vi "非均匀ADC.vi"(0 "输入的模拟信号取样值 V":dbl=2.56, 3 "Vref V":dbl=2.56) -> (7 "数字编码":i32[](array[numeric]))   [LabVIEW 2020]
panel:
  out "Numeric":i32
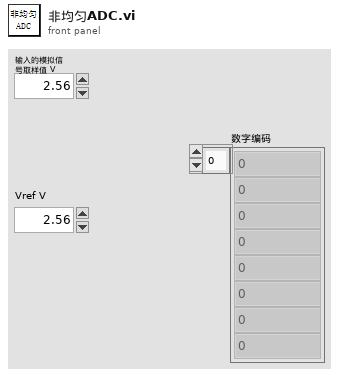
[diagram p1: front panel]
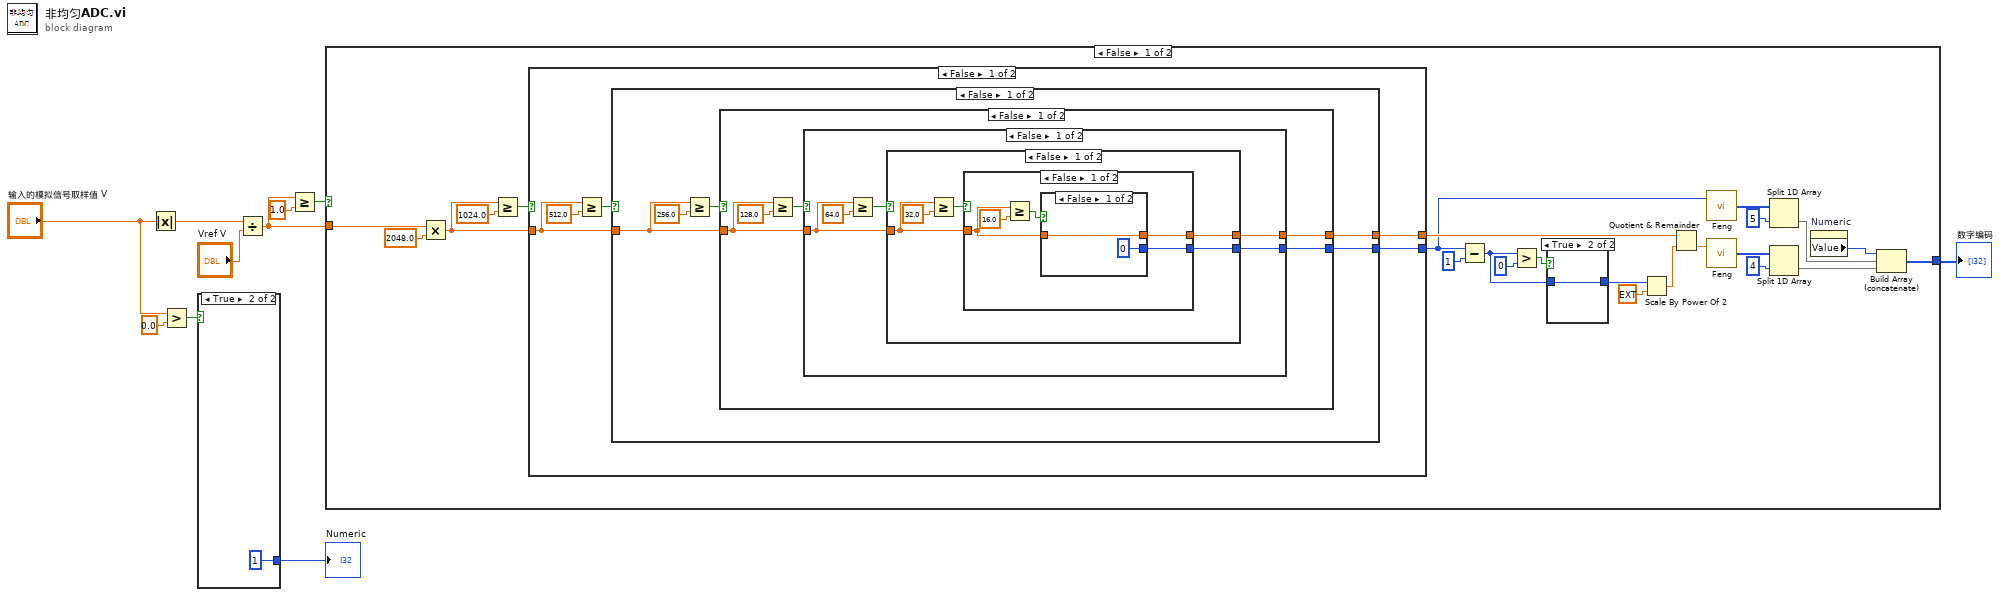
[diagram p0: block diagram]
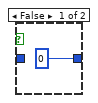
[diagram p2: hidden frame]
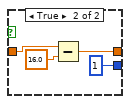
[diagram p3: hidden frame]
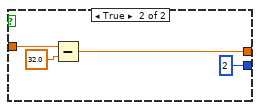
[diagram p4: hidden frame]
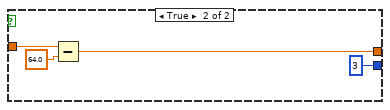
[diagram p5: hidden frame]
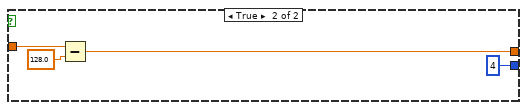
[diagram p6: hidden frame]
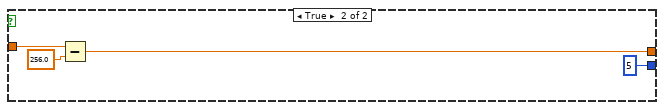
[diagram p7: hidden frame]
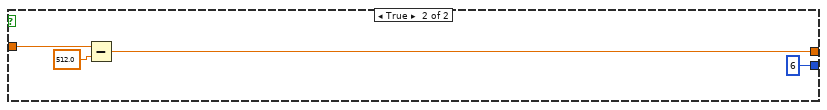
[diagram p8: hidden frame]
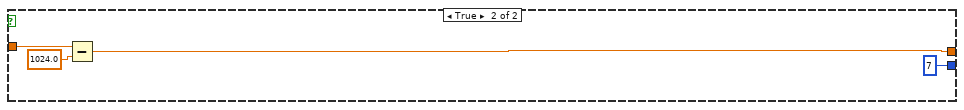
[diagram p9: hidden frame]
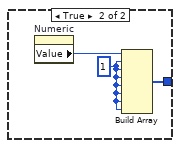
[diagram p10: hidden frame]
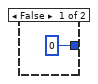
[diagram p11: hidden frame]
diagram:
  n1 = Absolute Value(x="输入的模拟信号取样值 V") -> (abs(x)=w8:dbl)
  n2 = Greater?(x="输入的模拟信号取样值 V", y=0.0) -> (0:w9:bool)
  n3 = case shown="True" w9 {
    tunnel: [0 1] -> w6
    frame False {
    }
    frame True {
    }
  }
  "Numeric" <- w6
  n4 = Divide(x=w8, y="Vref V") -> (x/y=w4:dbl)
  n5 = Greater Or Equal?(x=w4, y=1.0) -> (x >= y?=w2:bool)
  n6 = case shown="False" w2 {
    tunnel: w4 -> [w20 _]
    tunnel: [w19 w98] -> w3
    frame False {
      n7 = Multiply(x=w20, y=2048.0) -> (x*y=w32:dbl)
      n8 = Greater Or Equal?(x=w32, y=1024.0) -> (x >= y?=w33:bool)
      n9 = case shown="False" w33 {
        tunnel: w32 -> [w40 w97]
        tunnel: [w39 w95] -> w26
        tunnel: [w38 7] -> w18
        frame False {
          n10 = Greater Or Equal?(x=w40, y=512.0) -> (x >= y?=w41:bool)
          n11 = case shown="False" w41 {
            tunnel: w40 -> [w45 w92]
            tunnel: [w44 6] -> w38
            tunnel: [w43 w90] -> w39
            frame False {
              n12 = Greater Or Equal?(x=w45, y=256.0) -> (x >= y?=w46:bool)
              n13 = case shown="False" w46 {
                tunnel: w45 -> [w49 w88]
                tunnel: [w48 w87] -> w43
                tunnel: [w50 5] -> w44
                frame False {
                  n14 = Greater Or Equal?(x=w49, y=128.0) -> (x >= y?=w51:bool)
                  n15 = case shown="False" w51 {
                    tunnel: [w55 4] -> w50
                    tunnel: w49 -> [w54 w83]
                    tunnel: [w53 w82] -> w48
                    frame False {
                      n16 = Greater Or Equal?(x=w54, y=64.0) -> (x >= y?=w56:bool)
                      n17 = case shown="False" w56 {
                        tunnel: [w60 3] -> w55
                        tunnel: w54 -> [w59 w80]
                        tunnel: [w58 w78] -> w53
                        frame False {
                          n18 = Greater Or Equal?(x=w59, y=32.0) -> (x >= y?=w61:bool)
                          n19 = case shown="False" w61 {
                            tunnel: [w65 2] -> w60
                            tunnel: w59 -> [w64 w76]
                            tunnel: [w63 w74] -> w58
                            frame False {
                              n20 = Greater Or Equal?(x=w64, y=16.0) -> (x >= y?=w66:bool)
                              n21 = case shown="False" w66 {
                                tunnel: [0 1] -> w65
                                tunnel: w64 -> [w68 w71]
                                tunnel: [w68 w70] -> w63
                                frame False {
                                }
                                frame True {
                                n22 = Subtract(x=w71, y=16.0) -> (x-y=w70:dbl)
                                }
                              }
                            }
                            frame True {
                              n23 = Subtract(x=w76, y=32.0) -> (x-y=w74:dbl)
                            }
                          }
                        }
                        frame True {
                          n24 = Subtract(x=w80, y=64.0) -> (x-y=w78:dbl)
                        }
                      }
                    }
                    frame True {
                      n25 = Subtract(x=w83, y=128.0) -> (x-y=w82:dbl)
                    }
                  }
                }
                frame True {
                  n26 = Subtract(x=w88, y=256.0) -> (x-y=w87:dbl)
                }
              }
            }
            frame True {
              n27 = Subtract(x=w92, y=512.0) -> (x-y=w90:dbl)
            }
          }
        }
        frame True {
          n28 = Subtract(x=w97, y=1024.0) -> (x-y=w95:dbl)
        }
      }
      n29 = Subtract(x=w18, y=1) -> (x-y=w14:i32)
      n30 = Greater?(x=w14, y=0) -> (0:w15:bool)
      n31 = case shown="True" w15 {
        tunnel: w14 -> [_ w37]
        tunnel: [0 w37] -> w13
        frame False {
        }
        frame True {
        }
      }
      n32 = Scale By Power Of 2(n=w13, x=ext 1.0) -> (x*2^n=w27:ext)
      n33 = Quotient & Remainder(x=w26, y=w27) -> (floor(x/y)=w17:ext)  [unwired: 1 out]
      n34 = call "Feng.vi"("decimal 2"=w18) -> ("bitstream 3"=w31:i32[])  [unwired: 1 in]
      n35 = call "Feng.vi"("decimal 2"=w17) -> ("bitstream 3"=w24:i32[])  [unwired: 1 in]
      n36 = Split 1D Array(array=w31, index=5) -> (second subarray=w21:i32[])  [unwired: 1 out]
      n37 = Split 1D Array(array=w24, index=4) -> (second subarray=w22:i32[])  [unwired: 1 out]
      n38 = property on="Numeric" class="DigNum (strict)"() -> ("Value"=w23:i32)  [unwired: 2 in, 2 out]
      n39 = Build Array (concatenate)(w23, w21, w22) -> (w19:i32[])
    }
    frame True {
      w99 = 1
      n40 = property on="Numeric" class="DigNum (strict)"() -> ("Value"=w100:i32)  [unwired: 2 in, 2 out]
      n41 = Build Array(w100, w99, w99, w99, w99, w99, w99, w99) -> (w98:i32[])
    }
  }
  "数字编码" <- w3
